vi "Popup - Event Log Viewer.vi"(8 "Error IN":errorcluster) -> (0 "Error OUT":errorcluster)   [LabVIEW 2018]
uses:
  <vilib>/Utility/miscctls.llb/LVRowAndColumnUnsignedTypeDef.ctl
  Globals/Global - Configuration Options.vi
  <vilib>/Utility/file.llb/Read Delimited Spreadsheet (string).vi
panel:
  in  "Export":bool
  in  "OK":bool=TRUE
  out "Event Log":string[][](table)
  # "*exports as .zip file"
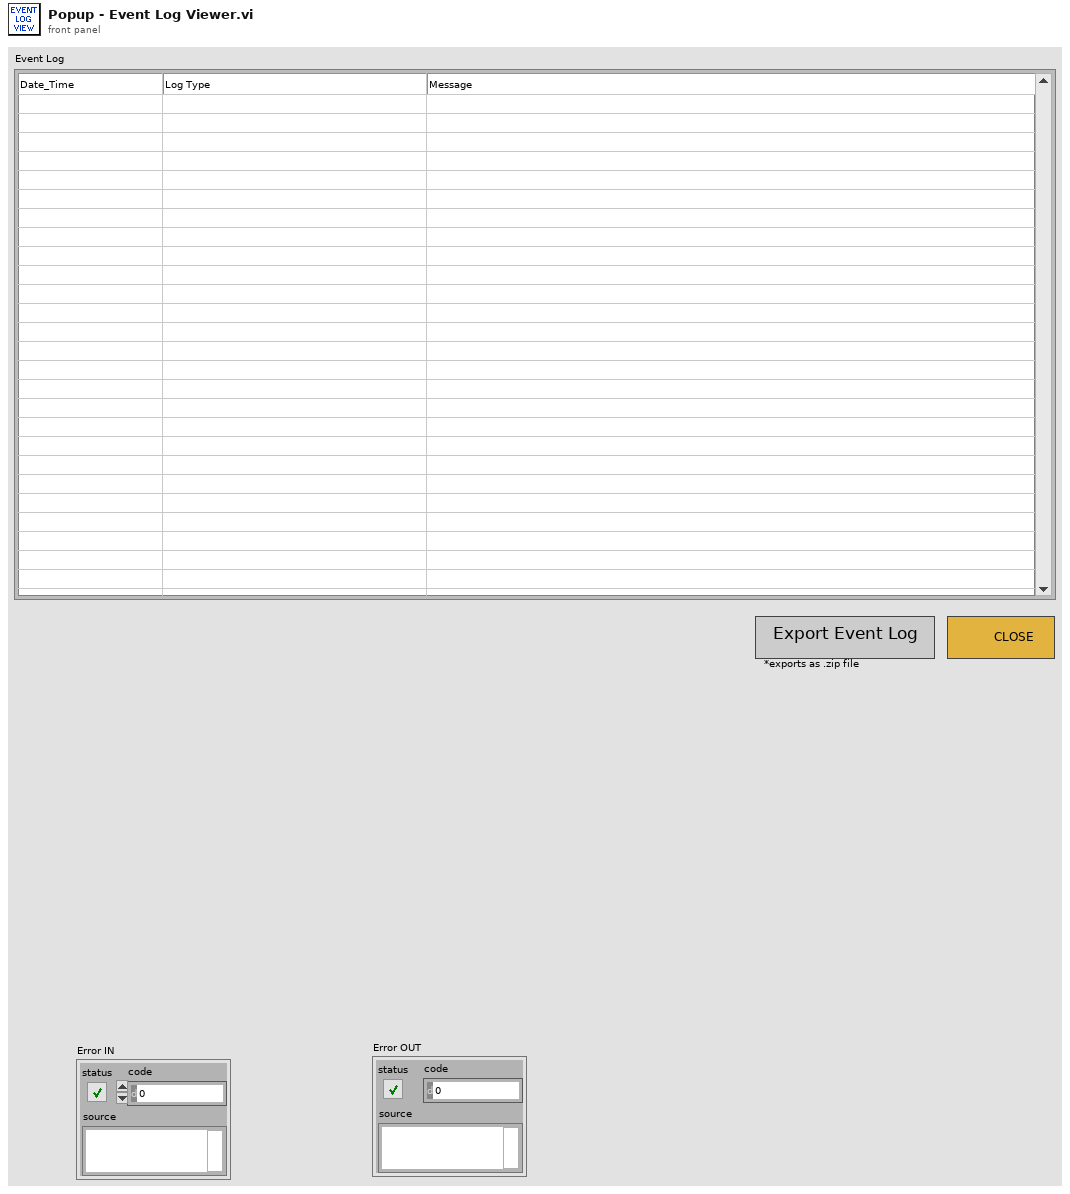
[diagram p1: front panel]
types:
  T1 = typedef "LVRowAndColumnUnsignedTypeDef.ctl" = cluster{"Row":u32, "Column":u32}
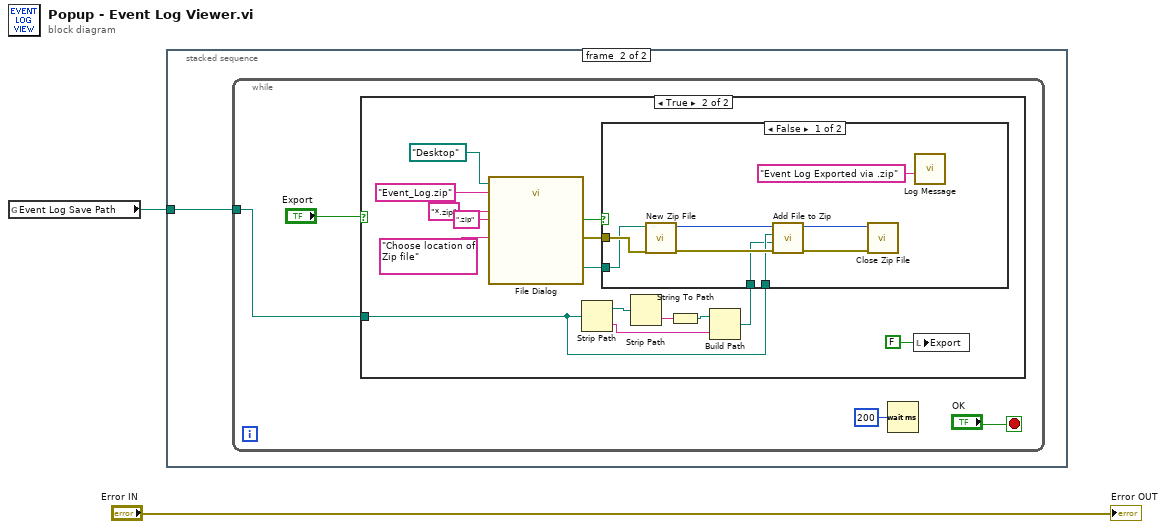
[diagram p0: block diagram]
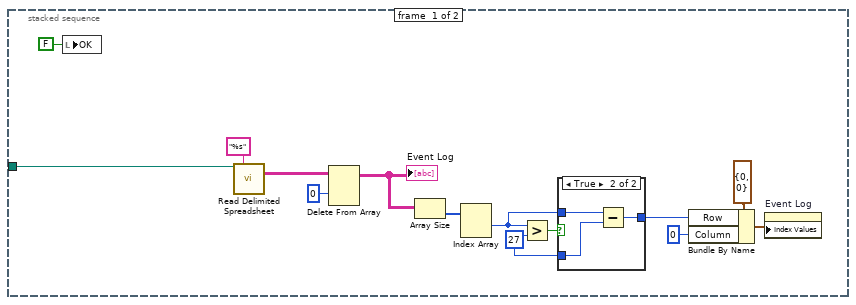
[diagram p2: hidden frame]
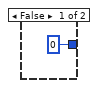
[diagram p3: hidden frame]
diagram:
  n1 = global read "Global - Configuration Options.vi" "Event Log Save Path"() -> (w1:path)
  n2 = stacked-sequence {
    tunnel: w1 -> [w3 w21]
    frame #0 {
      w11 = 27 ("y")
      n3 = local write "OK"(FALSE ("OK")) -> ()
      n4 = call-poly <vilib>:"Read Delimited Spreadsheet.vi"("file path (dialog if empty)"=w3, "format (%s)"="%s" ("format (%.3f)")) -> ("all rows"=w9:string[][])  [unwired: 8 in, 5 out]
      n5 = Delete From Array(array=w9, index (row)=0) -> (array with subset deleted=w8:string[][])  [unwired: 2 in, 1 out]
      "Event Log" <- w8
      n6 = Array Size(array=w8) -> (size(s)=w14:i32[])
      n7 = Index Array(array=w14) -> (element #1=w12:i32)  [unwired: 2 in, 1 out]
      n8 = Greater?(x=w12, y=w11) -> (0:w13:bool)
      n9 = case shown="True" w13 {
        tunnel: w12 -> [_ w20]
        tunnel: w11 -> [_ w19]
        tunnel: [0 w18] -> w4
        frame False {
        }
        frame True {
          n10 = Subtract(x=w20, y=w19) -> (x-y=w18:i32)
        }
      }
      n11 = Bundle By Name(cluster=T1 {"Row"=0, "Column"=0} ("Index Values"), "Row"=w4, "Column"=u32 0) -> (w6:T1)
      n12 = property on="Event Log" class="Tbl (strict)"("Index Values"=w6) -> ()  [unwired: 2 in, 2 out]
    }
    frame #1 {
      n13 = while {
        tunnel: w21 -> [w22]
        stop <- "OK" stop-if-true
        n14 = case shown="True" "Export" {
          tunnel: w22 -> [_ w26]
          frame False {
          }
          frame True {
            n15 = call "File Dialog"("start path"=path "Desktop", "prompt"="Choose location of Zip file", "default name"="Event_Log.zip", "pattern (all files)"="*.zip", "pattern label"=".zip") -> ("selected path"=w34:path, "cancelled"=w28:bool, "error out"=w35:errorcluster)  [unwired: 7 in, 1 out]
            n16 = Strip Path(path=w26) -> (stripped path=w33:path, name=w30:string)
            n17 = Strip Path(path=w33) -> (name=w32:string)  [unwired: 1 out]
            n18 = String To Path(string=w32) -> (path=w31:path)
            n19 = Build Path(base path=w31, name or relative path=w30) -> (appended path=w29:path)
            n20 = case shown="False" w28 {
              tunnel: w35 -> [w45 _]
              tunnel: w34 -> [w44 _]
              tunnel: w26 -> [w43 _]
              tunnel: w29 -> [w42 _]
              frame False {
                n21 = call <vilib>:"New Zip File.vi"("error in (no error)"=w45, "target"=w44) -> ("error out"=w48:errorcluster, "zip file out"=w46:i64)  [unwired: 3 in, 1 out]
                n22 = call <vilib>:"Add File to Zip.vi"("error in (no error)"=w48, "destination path in zip"=w42, "source file path"=w43, "zip file in"=w46) -> ("error out"=w49:errorcluster, "zip file out"=w47:i64)  [unwired: 6 in]
                n23 = call <vilib>:"Close Zip File.vi"("error in (no error)"=w49, "zip file in"=w47) -> ()  [unwired: 5 in, 1 out]
                n24 = call "Log Message.vi"("Message"="Event Log Exported via .zip") -> ()  [unwired: 9 in, 2 out]
              }
              frame True {
              }
            }
            n25 = local write "Export"(FALSE ("OK Button")) -> ()
          }
        }
        n26 = Wait (ms)(milliseconds to wait=u32 200) -> ()  [unwired: 1 out]
      }
    }
  }
  "Error OUT" <- "Error IN"
